vi "LN.pump.vi"(7 "error in (no error)":errorcluster, 8 "Auto (on) /Manual (off)":bool, 9 "0-30":u8, 10 "VISA resource name":refnum<visa-resource-name>) -> (0 "error out":errorcluster, 3 "VISA resource name out":refnum<visa-resource-name>)   [LabVIEW 8.6]
panel:
  out "concatenated string":string
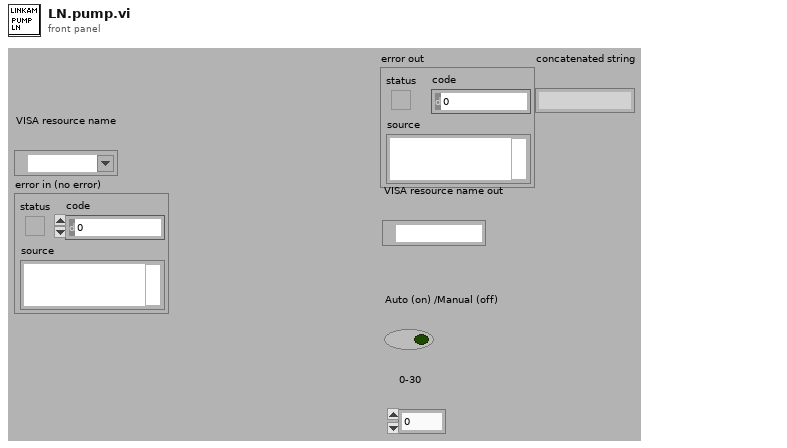
[diagram p1: front panel]
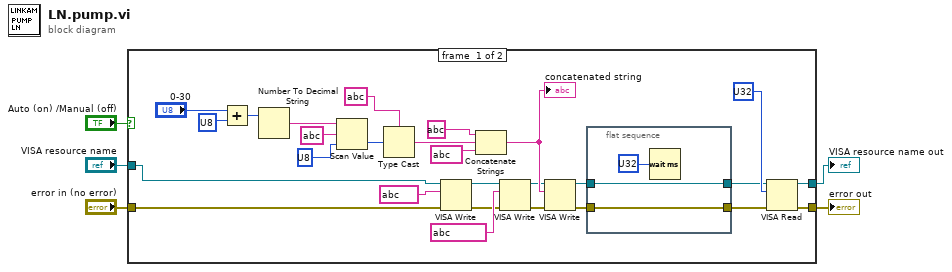
[diagram p0: block diagram]
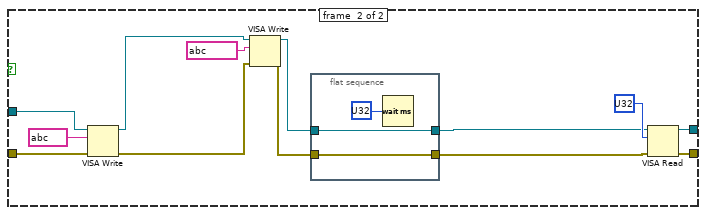
[diagram p2: hidden frame]
diagram:
  n1 = case shown="True" "Auto (on) /Manual (off)" {
    tunnel: "VISA resource name" -> [w14 w44]
    tunnel: "error in (no error)" -> [w12 w43]
    tunnel: [w31 w48] -> w2
    tunnel: [w32 w47] -> w1
    frame #0 {
      n2 = Add(x="0-30", y=u8 ?) -> (x+y=w21:u8)
      n3 = Number To Decimal String(number=w21) -> (decimal integer string=w20:string)  [unwired: 1 in]
      n4 = Scan Value(string=w20, format string=string ?, default (0 dbl)=u8 ?) -> (value=w15:u8)  [unwired: 1 out]
      n5 = Type Cast(type=string ?, x=w15) -> (*(type *) &x=w16:string)
      n6 = VISA Write(VISA resource name=w14, write buffer=string ?, error in (no error)=w12) -> (VISA resource name out=w13:refnum<visa-resource-name>, error out=w11:errorcluster)  [unwired: 1 out]
      n7 = Concatenate Strings(string ? ("string"), w16, string ? ("string")) -> (w27:string)
      "concatenated string" <- w27
      n8 = VISA Write(VISA resource name=w13, write buffer=string ?, error in (no error)=w11) -> (VISA resource name out=w24:refnum<visa-resource-name>, error out=w23:errorcluster)  [unwired: 1 out]
      n9 = VISA Write(VISA resource name=w24, write buffer=w27, error in (no error)=w23) -> (VISA resource name out=w9:refnum<visa-resource-name>, error out=w8:errorcluster)  [unwired: 1 out]
      n10 = flat-sequence {
        tunnel: w9 -> [w34]
        tunnel: [w34] -> w6
        tunnel: w8 -> [w33]
        tunnel: [w33] -> w7
        frame #0 {
          n11 = Wait (ms)(milliseconds to wait=u32 ?) -> ()  [unwired: 1 out]
        }
      }
      n12 = VISA Read(VISA resource name=w6, byte count=u32 ?, error in (no error)=w7) -> (VISA resource name out=w31:refnum<visa-resource-name>, error out=w32:errorcluster)  [unwired: 2 out]
    }
    frame #1 {
      n13 = VISA Write(VISA resource name=w44, write buffer=string ?, error in (no error)=w43) -> (VISA resource name out=w38:refnum<visa-resource-name>, error out=w39:errorcluster)  [unwired: 1 out]
      n14 = VISA Write(VISA resource name=w38, write buffer=string ?, error in (no error)=w39) -> (VISA resource name out=w37:refnum<visa-resource-name>, error out=w36:errorcluster)  [unwired: 1 out]
      n15 = flat-sequence {
        tunnel: w37 -> [w50]
        tunnel: [w50] -> w41
        tunnel: w36 -> [w49]
        tunnel: [w49] -> w40
        frame #0 {
          n16 = Wait (ms)(milliseconds to wait=u32 ?) -> ()  [unwired: 1 out]
        }
      }
      n17 = VISA Read(VISA resource name=w41, byte count=u32 ?, error in (no error)=w40) -> (VISA resource name out=w48:refnum<visa-resource-name>, error out=w47:errorcluster)  [unwired: 2 out]
    }
  }
  "error out" <- w1
  "VISA resource name out" <- w2
